vi "CSV_Image_Data_Append_2.0.vi"(0 "Data":T1={"Camera 1"={"Camera1"="", "Cam 1"=FALSE, "CAM1 Model"=enum."a2A5328-15ucBAS", "Cam1 ID"=0}, "Camera 2"={"Camera2"="", "Cam 2"=FALSE, "CAM2 Model"=enum."a2A5328-15ucBAS", "Cam2 ID"=0}, "Image"={"Camera1_Img"=refnum, "Camera2_Img"=refnum, "Img1_Orig_Disp"=refnum, "Img2_Orig_Disp"=refnum, "Img1_Orig_RGB"=refnum, "Img2_Orig_RGB"=refnum, "Blue_Plane_Extract"=refnum, "Subtracted_Plane"=refnum, "Img1_Binary"=refnum, "Img2_Binary"=refnum, "Crop_Mask"=refnum, "Img1_Save"=refnum, "Img2_Save"=refnum, "Img1_Cali_Full"=refnum, "Img2_Cali_Full"=refnum, "Img1_Cali_Detect"=refnum, "Img2_Cali_Detect"=refnum}, "Ques"={"Cam 1 queue"=refnum, "Cam 2 queue"=refnum, "Cam 1 - save queue"=refnum, "Cam 2 - save queue"=refnum, "Image Process Queue Size"=500, "Image Save Queue Size"=500, "Overload threshold"=500, "Max large object threshold"=0}, "Arduino SRS"={"Pinch-valve"="", "Actuator"=FALSE, "Arduino Uno"="", "Valve state"=enum."Open"}, "Pump"={"Port"="", "Connection"=FALSE, "Flush Size"=0, "Command"="", "Pump Size"=enum."None", "Pump"="", "Ready"=FALSE}, "Camera settings"={"Detection settings"={"Sample size threshold"=500, "Detection Region %"=30.0, "Timeout Sample"=200}, "Lens/camera settings"={"Aperture"=enum."Item 0", "Legacy Cam Attributes"=FALSE, "Max Framerate"=100, "Exposure Time"=1000.0, "Framerate"=15}, "Crop settings"={"Cam1"={"Rectangle 1"={"Left"=0, "Top"=0, "Right"=0, "Bottom"=0, "Rotation"=0.0}, "Camera Orientation 1"="", "Pixel to mm 1"=0.0}, "Cam2"={"Rectangle 2"={"Left"=0, "Top"=0, "Right"=0, "Bottom"=0, "Rotation"=0.0}, "Camera Orientation 2"="", "Pixel to mm 2"=0.0}}}, "Arduino ISS"={"Mega F3"="", "Phase3"=FALSE, "Barcode"="", "Sorting sys."=FALSE, "Initial size"=0.0, "Size Interval"=0.0, "Mun. of containers"=0.0, "Container nr."=0.0, "Arduino Mega"="", "Attempts"=0.0}, "Img_Capt"=FALSE, "Empty_Refill"=FALSE, "I don't think is in use"={"Light intensity"=100}, "Extended setup"={"Location"="Station", "Latitude"="Station", "Longitude"="Station", "Determiner"="Station", "Sex"="Station", "Station"="", "Collection date"=""}, "Main interface"={"Sample Name"="Test Sample", "Operator"="JFR", "Species Name"="", "Other Notes"=""}, "Tap1"=0, "SystemVersion"=0, "System Serial"="", "Exit"=FALSE, "Kuvette Full"=FALSE, "Core JKI"={"Current VI Reference"=refnum, "Close Panel on Exit?"=FALSE}, "Calibration"={"Calibration 1"=path "C:/Users/au540322/Desktop/IHS_Project/images/Debris/Debris_0/Debris_0_2019_06_01-23-32-49-686.PNG", "Calibration 2"=path "C:/Users/au540322/Desktop/IHS_Project/images/Debris/Debris_0/Debris_0_2019_06_01-23-32-49-686.PNG", "Detect 1"=path "C:/Users/au540322/Desktop/IHS_Project/images/Debris/Debris_0/Debris_0_2019_06_01-23-32-49-686.PNG", "Detect 2"=path "C:/Users/au540322/Desktop/IHS_Project/images/Debris/Debris_0/Debris_0_2019_06_01-23-32-49-686.PNG"}, "Auto Flush"=FALSE, "Status History"="", "Timestamp Start"=""} {"SystemVersion" items=["Standard", "XL"]; "Tap1" items=["Session Data", "Extended Setup", "Buffer", "Camera", "Dispenser", "Stats", "Connections"]; "I don't think is in use"."Light intensity" scale=0.0..100.0; "Camera settings"."Crop settings"."Cam2"."Rectangle 2"."Rotation" format="%.2f"; "Camera settings"."Crop settings"."Cam2"."Rectangle 2"."Left" scale=0.0..1024.0; "Camera settings"."Crop settings"."Cam2"."Rectangle 2"."Right" scale=0.0..1024.0; "Camera settings"."Crop settings"."Cam1"."Rectangle 1"."Rotation" format="%.2f"; "Camera settings"."Crop settings"."Cam1"."Rectangle 1"."Left" scale=0.0..1024.0; "Camera settings"."Crop settings"."Cam1"."Rectangle 1"."Right" scale=0.0..1024.0; "Camera settings"."Lens/camera settings"."Framerate" min=1; "Camera settings"."Lens/camera settings"."Max Framerate" min=1; "Camera settings"."Detection settings"."Sample size threshold" min=1; "Pump"."Flush Size" min=0 max=6000 step=100; "Ques"."Overload threshold" min=1; "Ques"."Image Save Queue Size" min=1; "Ques"."Image Process Queue Size" min=1}, 1 "Image path":string, 2 "Sample Name":string, 3 "Image Name":string, 4 "Sample Data":dbl[](array[numeric]), 5 "ROI Descriptor":T5, 7 "Timestamp":string) -> ()   [LabVIEW 2024]
uses:
  controls/Data_JKI.ctl
  <vilib>/userDefined/High Color/IMAQdx.ctl
  <vilib>/vision/Image Controls.llb/IMAQ Image.ctl
  <vilib>/Utility/file.llb/Write Delimited Spreadsheet (string).vi
panel:
  out "string":string
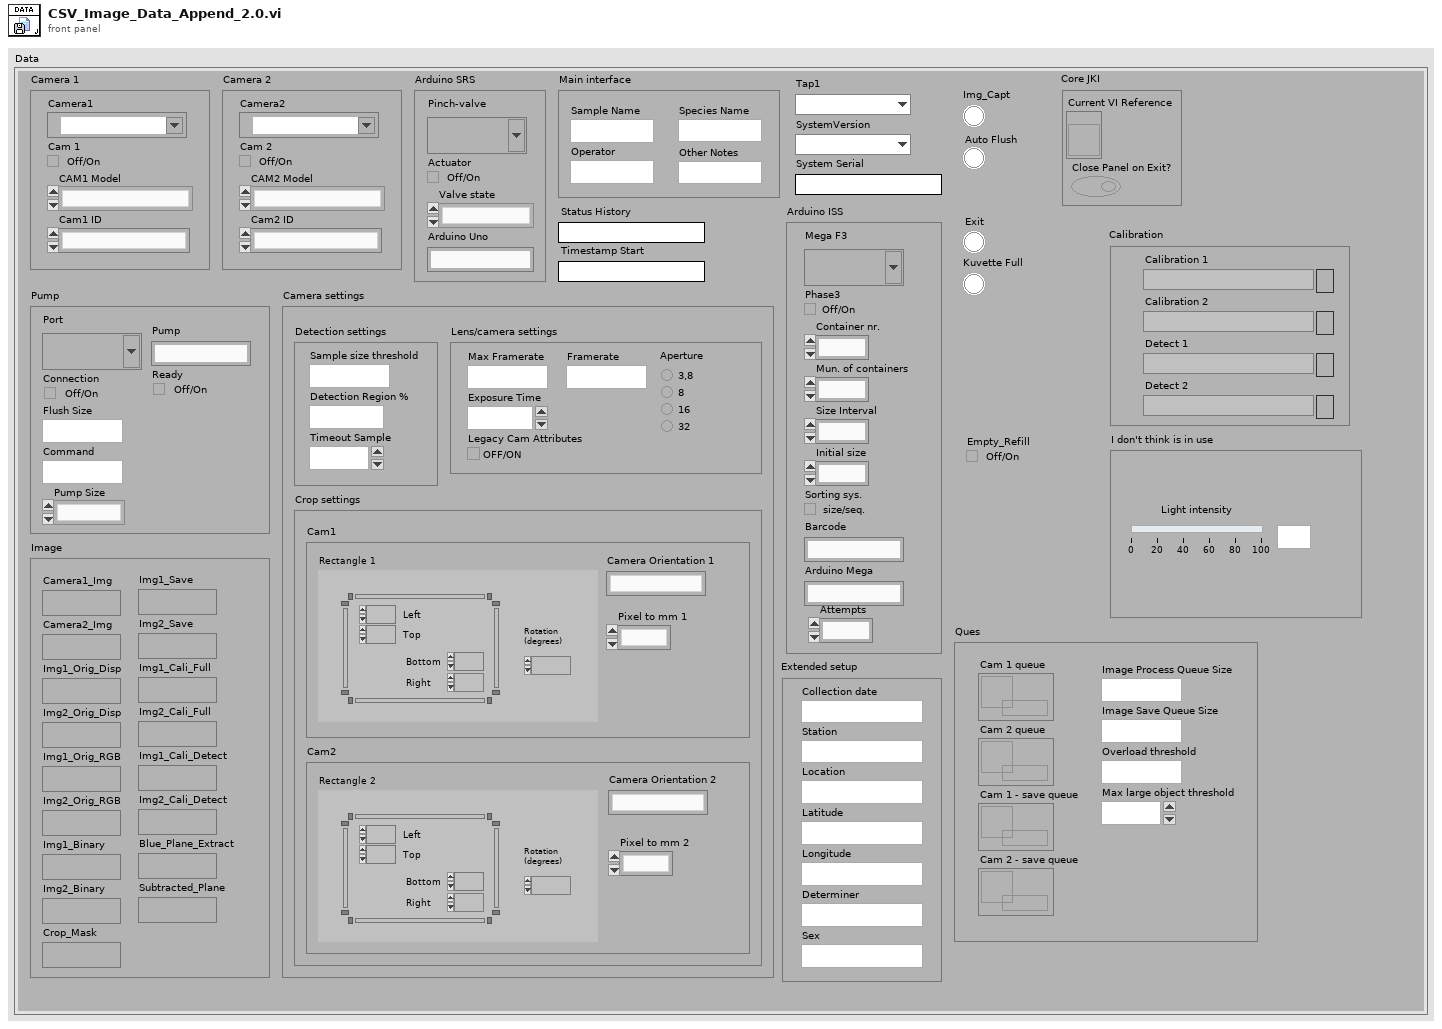
[diagram p1: front panel]
types:
  T1 = typedef "Data_JKI.ctl" = cluster{"Camera 1":cluster{"Camera1":T2, "Cam 1":bool, "CAM1 Model":enum16{"a2A5328-15ucBAS", "acA1920-155uc"}, "Cam1 ID":i32}, "Camera 2":cluster{"Camera2":T2, "Cam 2":bool, "CAM2 Model":enum16{"a2A5328-15ucBAS", "acA1920-155uc"}, "Cam2 ID":i32}, "Image":cluster{"Camera1_Img":T3, "Camera2_Img":T3, "Img1_Orig_Disp":T3, "Img2_Orig_Disp":T3, "Img1_Orig_RGB":T3, "Img2_Orig_RGB":T3, "Blue_Plane_Extract":T3, "Subtracted_Plane":T3, "Img1_Binary":T3, "Img2_Binary":T3, "Crop_Mask":T3, "Img1_Save":T3, "Img2_Save":T3, "Img1_Cali_Full":T3, "Img2_Cali_Full":T3, "Img1_Cali_Detect":T3, "Img2_Cali_Detect":T3}, "Ques":cluster{"Cam 1 queue":refnum<queue>, "Cam 2 queue":refnum<queue>, "Cam 1 - save queue":refnum<queue>, "Cam 2 - save queue":refnum<queue>, "Image Process Queue Size":i32, "Image Save Queue Size":i32, "Overload threshold":i32, "Max large object threshold":i32}, "Arduino SRS":cluster{"Pinch-valve":refnum<visa-resource-name>, "Actuator":bool, "Arduino Uno":string, "Valve state":enum16{"Standby", "Close", "Open"}}, "Pump":cluster{"Port":refnum<visa-resource-name>, "Connection":bool, "Flush Size":i32, "Command":string, "Pump Size":enum16{"None", "Small", "Large"}, "Pump":string, "Ready":bool}, "Camera settings":cluster{"Detection settings":cluster{"Sample size threshold":i32, "Detection Region %":dbl, "Timeout Sample":i32}, "Lens/camera settings":cluster{"Aperture":enum32{"Item 0", "Item 1", "Item 2", "Item 3"}, "Legacy Cam Attributes":bool, "Max Framerate":i32, "Exposure Time":dbl, "Framerate":i32}, "Crop settings":cluster{"Cam1":cluster{"Rectangle 1":T4, "Camera Orientation 1":string, "Pixel to mm 1":dbl}, "Cam2":cluster{"Rectangle 2":T4, "Camera Orientation 2":string, "Pixel to mm 2":dbl}}}, "Arduino ISS":cluster{"Mega F3":refnum<visa-resource-name>, "Phase3":bool, "Barcode":string, "Sorting sys.":bool, "Initial size":dbl, "Size Interval":dbl, "Mun. of containers":dbl, "Container nr.":dbl, "Arduino Mega":string, "Attempts":dbl}, "Img_Capt":bool, "Empty_Refill":bool, "I don't think is in use":cluster{"Light intensity":i32}, "Extended setup":cluster{"Location":string, "Latitude":string, "Longitude":string, "Determiner":string, "Sex":string, "Station":string, "Collection date":string}, "Main interface":cluster{"Sample Name":string, "Operator":string, "Species Name":string, "Other Notes":string}, "Tap1":u16, "SystemVersion":u16, "System Serial":string, "Exit":bool, "Kuvette Full":bool, "Core JKI":cluster{"Current VI Reference":refnum<vi>, "Close Panel on Exit?":bool}, "Calibration":cluster{"Calibration 1":path, "Calibration 2":path, "Detect 1":path, "Detect 2":path}, "Auto Flush":bool, "Status History":string, "Timestamp Start":string}
  T2 = typedef "IMAQdx.ctl" = refnum<k21>
  T3 = typedef "IMAQ Image.ctl" = refnum<image>
  T4 = typedef "IMAQ Rectangle" = cluster{"Left":i32, "Top":i32, "Right":i32, "Bottom":i32, "Rotation":dbl}
  T5 = cluster{"Global Rectangle":i32[], "Contours":cluster{"ID":enum32{"External", "Internal"}, "Type":u32, "Coordinates":i32[]}[]}
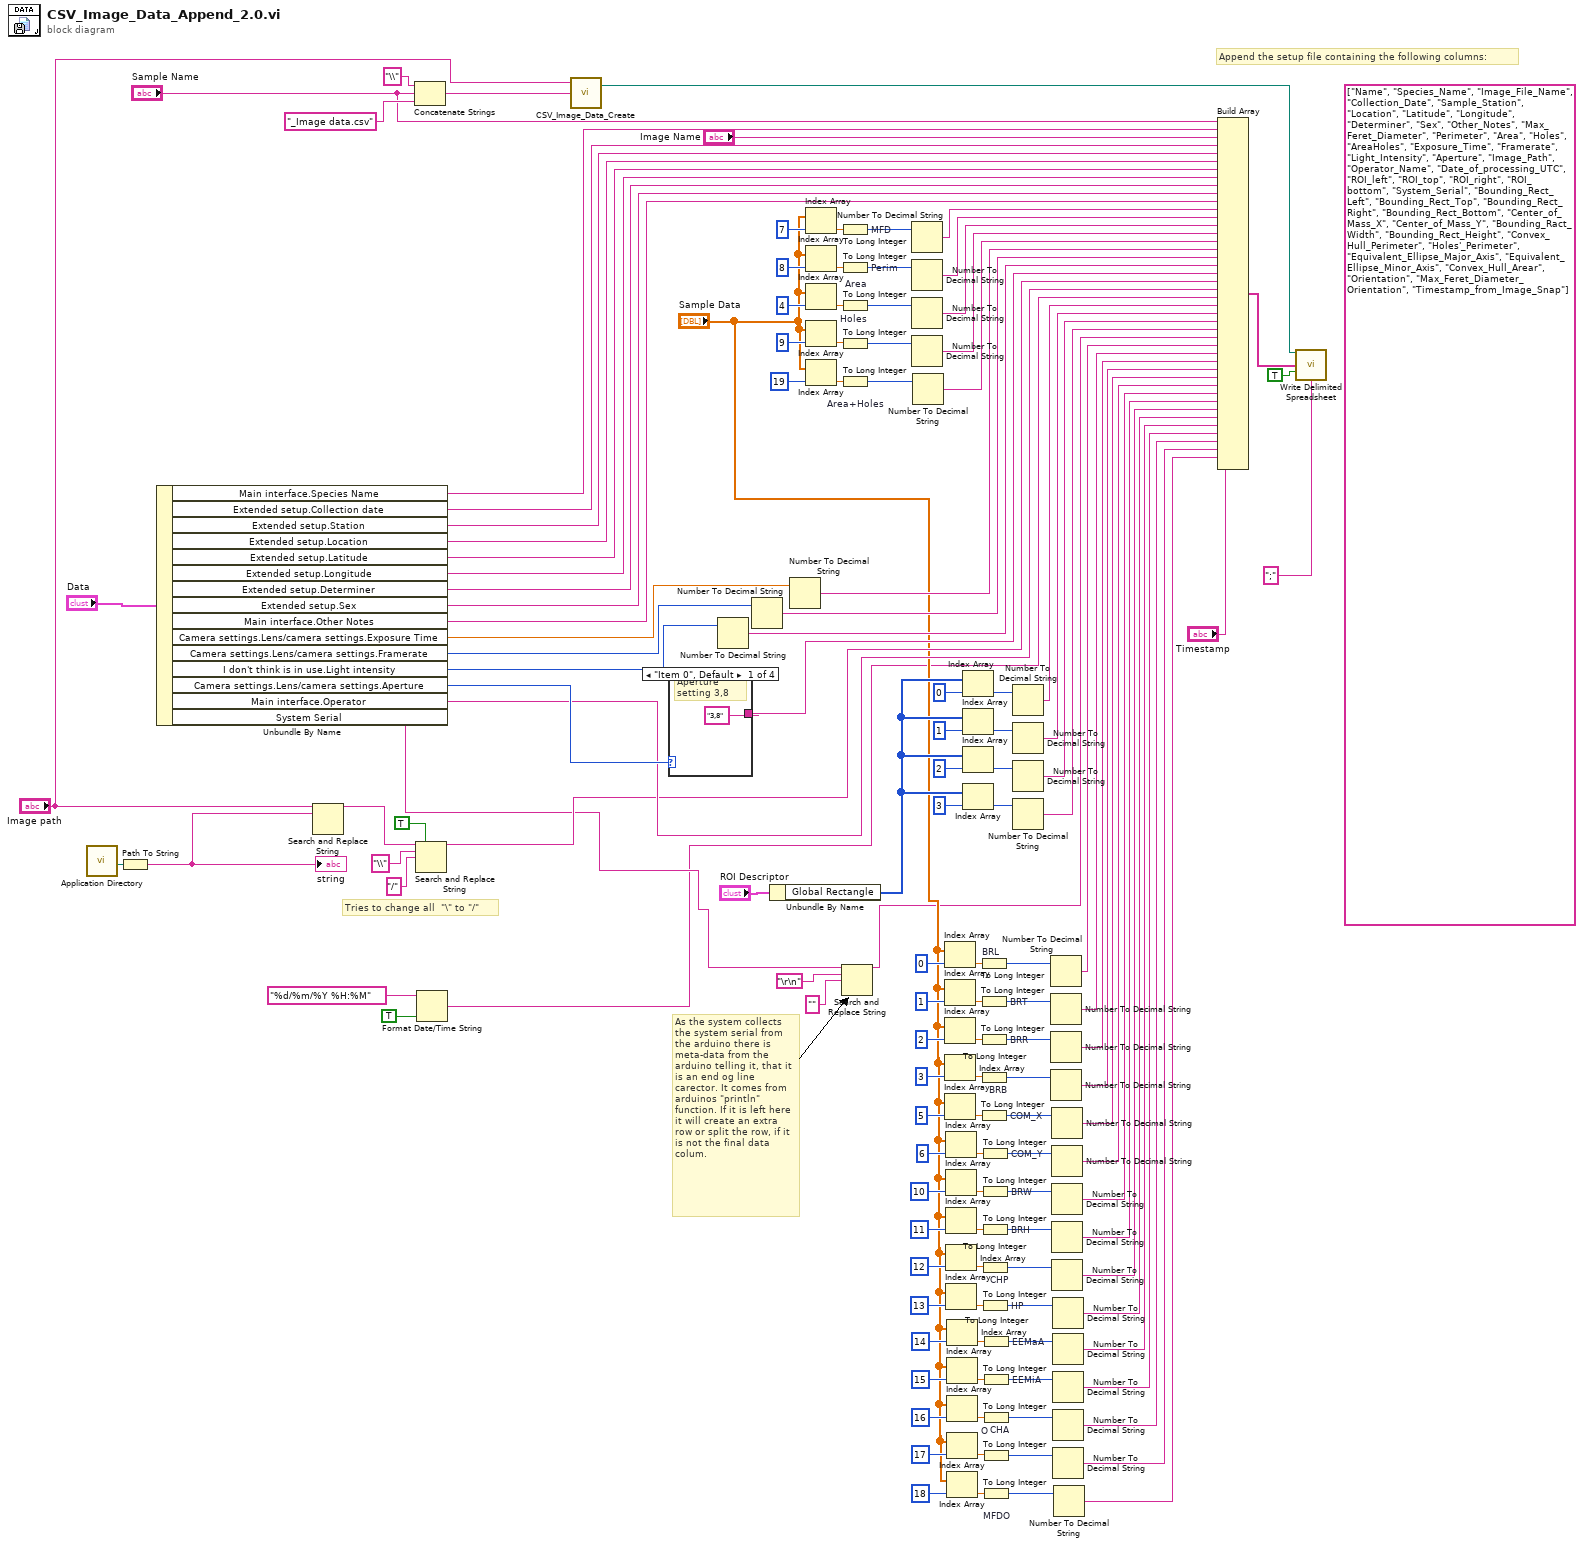
[diagram p0: block diagram]
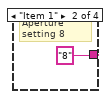
[diagram p2: hidden frame]
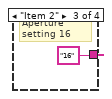
[diagram p3: hidden frame]
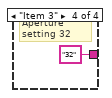
[diagram p4: hidden frame]
diagram:
  (unwired) string[] ["Name", "Species_Name", "Image_File_Name", "Collection_Date", "Sample_Station", "Location", "Latitude", "Longitude", "Determiner", "Sex", "Other_Notes", "Max_Feret_Diameter", "Perimeter", "Area", "Holes", "AreaHoles", "Exposure_Time", "Framerate", "Light_Intensity", "Aperture", "Image_Path", "Operator_Name", "Date_of_processing_UTC", "ROI_left", "ROI_top", "ROI_right", "ROI_bottom", "System_Serial", "Bounding_Rect_Left", "Bounding_Rect_Top", "Bounding_Rect_Right", "Bounding_Rect_Bottom", "Center_of_Mass_X", "Center_of_Mass_Y", "Bounding_Ract_Width", "Bounding_Rect_Height", "Convex_Hull_Perimeter", "Holes'_Perimeter", "Equivalent_Ellipse_Major_Axis", "Equivalent_Ellipse_Minor_Axis", "Convex_Hull_Arear", "Orientation", "Max_Feret_Diameter_Orientation", "Timestamp_from_Image_Snap"]
  # "As the system collects the system serial from the arduino there is meta-data from the arduino telling it, that it is an end og line carector. It comes from arduinos \"println\" function. If it is left here it will create an extra row or split the row, if it is not the final data colum."
  # "Tries to change all  \"\\\" to \"/\""
  # "Append the setup file containing the following columns:"
  n1 = call <vilib>:"Application Directory.vi"() -> ("Application Directory"=w136:path)
  n2 = Path To String(path=w136) -> (string=w135:string)
  "string" <- w135
  n3 = Unbundle By Name("Data") -> ("Main interface.Species Name"=w118:string, "Extended setup.Collection date"=w119:string, "Extended setup.Station"=w120:string, "Extended setup.Location"=w121:string, "Extended setup.Latitude"=w122:string, "Extended setup.Longitude"=w123:string, "Extended setup.Determiner"=w124:string, "Extended setup.Sex"=w125:string, "Main interface.Other Notes"=w126:string, "Camera settings.Lens/camera settings.Exposure Time"=w134:dbl, "Camera settings.Lens/camera settings.Framerate"=w81:i32, "I don't think is in use.Light intensity"=w133:i32, "Camera settings.Lens/camera settings.Aperture"=w132:enum32{"Item 0", "Item 1", "Item 2", "Item 3"}, "Main interface.Operator"=w127:string, "System Serial"=w22:string)
  n4 = Search and Replace String(input string="Image path", search string=w135) -> (result string=w69:string)  [unwired: 6 in, 3 out]
  n5 = Concatenate Strings("\\" ("string"), "Sample Name", "_Image data.csv") -> (w76:string)
  n6 = Search and Replace String(replace all?=TRUE ("replace all? (F)"), input string=w69, search string="\\", replace string="/" ("replace string (\"\")")) -> (result string=w70:string)  [unwired: 4 in, 3 out]
  n7 = Format Date/Time String(time format string (%c)="%d/%m/%Y %H:%M", UTC format=TRUE) -> (date/time string=w3:string)  [unwired: 1 in]
  n8 = call "CSV_Image_Data_Create.vi"("File name"=w76, "Image path"="Image path") -> ("Image data file"=w75:path)  [unwired: 2 in, 1 out]
  n9 = case shown="\"Item 0\", Default" w132 {
    tunnel: ["3,8" "8" "16" "32"] -> w128
    frame "Item 0", Default {
      # "Aperture setting 3,8"
    }
    frame "Item 1" {
      # "Aperture setting 8"
    }
    frame "Item 2" {
      # "Aperture setting 16"
    }
    frame "Item 3" {
      # "Aperture setting 32"
    }
  }
  n10 = Number To Decimal String(number=w133) -> (decimal integer string=w129:string)  [unwired: 1 in]
  n11 = Number To Decimal String(number=w81) -> (decimal integer string=w130:string)  [unwired: 1 in]
  n12 = Unbundle By Name("ROI Descriptor") -> ("Global Rectangle"=w86:i32[])
  n13 = Number To Decimal String(number=w134) -> (decimal integer string=w131:string)  [unwired: 1 in]
  n14 = Index Array ("MFD")(array="Sample Data", index=7) -> (element=w110:dbl)
  n15 = Index Array ("MFD")(array="Sample Data", index=8) -> (element=w105:dbl)
  n16 = Index Array ("MFD")(array="Sample Data", index=4) -> (element=w103:dbl)
  n17 = Index Array ("MFD")(array="Sample Data", index=9) -> (element=w104:dbl)
  n18 = Index Array ("MFD")(array="Sample Data", index=19) -> (element=w102:dbl)
  n19 = To Long Integer "MFD"(number=w110) -> (32bit integer=w116:i32)
  n20 = To Long Integer "Perim"(number=w105) -> (32bit integer=w115:i32)
  n21 = To Long Integer "Area"(number=w103) -> (32bit integer=w114:i32)
  n22 = To Long Integer "Holes"(number=w104) -> (32bit integer=w113:i32)
  n23 = To Long Integer "Area+Holes"(number=w102) -> (32bit integer=w112:i32)
  n24 = Search and Replace String(input string=w22, search string="\r\n", replace string="" ("replace string (\"\")")) -> (result string=w19:string)  [unwired: 5 in, 3 out]
  n25 = Number To Decimal String(number=w116) -> (decimal integer string=w101:string)  [unwired: 1 in]
  n26 = Number To Decimal String(number=w115) -> (decimal integer string=w100:string)  [unwired: 1 in]
  n27 = Number To Decimal String(number=w114) -> (decimal integer string=w99:string)  [unwired: 1 in]
  n28 = Number To Decimal String(number=w113) -> (decimal integer string=w98:string)  [unwired: 1 in]
  n29 = Number To Decimal String(number=w112) -> (decimal integer string=w97:string)  [unwired: 1 in]
  n30 = Index Array ("MFD")(array="Sample Data", index=0) -> (element=w62:dbl)
  n31 = Index Array ("MFD")(array="Sample Data", index=1) -> (element=w57:dbl)
  n32 = Index Array ("MFD")(array="Sample Data", index=2) -> (element=w55:dbl)
  n33 = Index Array ("MFD")(array="Sample Data", index=3) -> (element=w56:dbl)
  n34 = Index Array ("MFD")(array="Sample Data", index=5) -> (element=w54:dbl)
  n35 = Index Array ("MFD")(array="Sample Data", index=6) -> (element=w47:dbl)
  n36 = Index Array ("MFD")(array="Sample Data", index=10) -> (element=w42:dbl)
  n37 = Index Array ("MFD")(array="Sample Data", index=11) -> (element=w40:dbl)
  n38 = Index Array ("MFD")(array="Sample Data", index=12) -> (element=w41:dbl)
  n39 = Index Array ("MFD")(array="Sample Data", index=13) -> (element=w39:dbl)
  n40 = Index Array ("MFD")(array="Sample Data", index=14) -> (element=w32:dbl)
  n41 = Index Array ("MFD")(array="Sample Data", index=15) -> (element=w27:dbl)
  n42 = Index Array ("MFD")(array="Sample Data", index=16) -> (element=w25:dbl)
  n43 = Index Array ("MFD")(array="Sample Data", index=17) -> (element=w26:dbl)
  n44 = Index Array ("MFD")(array="Sample Data", index=18) -> (element=w24:dbl)
  n45 = Index Array ("MFD")(array=w86, index=0) -> (element=w94:i32)
  n46 = Index Array ("MFD")(array=w86, index=1) -> (element=w93:i32)
  n47 = Index Array ("MFD")(array=w86, index=2) -> (element=w92:i32)
  n48 = Index Array ("MFD")(array=w86, index=3) -> (element=w91:i32)
  n49 = To Long Integer "BRL"(number=w62) -> (32bit integer=w68:i32)
  n50 = To Long Integer "BRT"(number=w57) -> (32bit integer=w67:i32)
  n51 = To Long Integer "BRR"(number=w55) -> (32bit integer=w66:i32)
  n52 = To Long Integer "BRB"(number=w56) -> (32bit integer=w65:i32)
  n53 = To Long Integer "COM_X"(number=w54) -> (32bit integer=w64:i32)
  n54 = To Long Integer "COM_Y"(number=w47) -> (32bit integer=w53:i32)
  n55 = To Long Integer "BRW"(number=w42) -> (32bit integer=w52:i32)
  n56 = To Long Integer "BRH"(number=w40) -> (32bit integer=w51:i32)
  n57 = To Long Integer "CHP"(number=w41) -> (32bit integer=w50:i32)
  n58 = To Long Integer "HP"(number=w39) -> (32bit integer=w49:i32)
  n59 = To Long Integer "EEMaA"(number=w32) -> (32bit integer=w38:i32)
  n60 = To Long Integer "EEMiA"(number=w27) -> (32bit integer=w37:i32)
  n61 = To Long Integer "CHA"(number=w25) -> (32bit integer=w36:i32)
  n62 = To Long Integer "O"(number=w26) -> (32bit integer=w35:i32)
  n63 = To Long Integer "MFDO"(number=w24) -> (32bit integer=w34:i32)
  n64 = Number To Decimal String(number=w94) -> (decimal integer string=w85:string)  [unwired: 1 in]
  n65 = Number To Decimal String(number=w93) -> (decimal integer string=w84:string)  [unwired: 1 in]
  n66 = Number To Decimal String(number=w92) -> (decimal integer string=w83:string)  [unwired: 1 in]
  n67 = Number To Decimal String(number=w91) -> (decimal integer string=w82:string)  [unwired: 1 in]
  n68 = Number To Decimal String(number=w68) -> (decimal integer string=w18:string)  [unwired: 1 in]
  n69 = Number To Decimal String(number=w67) -> (decimal integer string=w17:string)  [unwired: 1 in]
  n70 = Number To Decimal String(number=w66) -> (decimal integer string=w16:string)  [unwired: 1 in]
  n71 = Number To Decimal String(number=w65) -> (decimal integer string=w15:string)  [unwired: 1 in]
  n72 = Number To Decimal String(number=w64) -> (decimal integer string=w14:string)  [unwired: 1 in]
  n73 = Number To Decimal String(number=w53) -> (decimal integer string=w13:string)  [unwired: 1 in]
  n74 = Number To Decimal String(number=w52) -> (decimal integer string=w12:string)  [unwired: 1 in]
  n75 = Number To Decimal String(number=w51) -> (decimal integer string=w11:string)  [unwired: 1 in]
  n76 = Number To Decimal String(number=w50) -> (decimal integer string=w10:string)  [unwired: 1 in]
  n77 = Number To Decimal String(number=w49) -> (decimal integer string=w9:string)  [unwired: 1 in]
  n78 = Number To Decimal String(number=w38) -> (decimal integer string=w8:string)  [unwired: 1 in]
  n79 = Number To Decimal String(number=w37) -> (decimal integer string=w7:string)  [unwired: 1 in]
  n80 = Number To Decimal String(number=w36) -> (decimal integer string=w6:string)  [unwired: 1 in]
  n81 = Number To Decimal String(number=w35) -> (decimal integer string=w5:string)  [unwired: 1 in]
  n82 = Number To Decimal String(number=w34) -> (decimal integer string=w4:string)  [unwired: 1 in]
  n83 = Build Array("Sample Name", w118, "Image Name", w119, w120, w121, w122, w123, w124, w125, w126, w101, w100, w99, w98, w97, w131, w130, w129, w128, w70, w127, w3, w85, w84, w83, w82, w19, w18, w17, w16, w15, w14, w13, w12, w11, w10, w9, w8, w7, w6, w5, w4, "Timestamp") -> (w117:string[])
  n84 = call-poly <vilib>:"Write Delimited Spreadsheet.vi"("file path (dialog if empty)"=w75, "1D data"=w117, "append to file? (new file:F)"=TRUE, "delimiter (\\t)"=";" ("delimiter (\\t)")) -> ()  [unwired: 10 in, 2 out]
